vi "提示信息.vi"(0 "LstBox引用句柄":refnum<vi>, 1 "截取数组大小":dbl, 2 "保留行数":dbl, 5 "旧信息":string[](array[string]), 7 "新信息":string, 11 "error in (no error)":errorcluster caption="错误输入（无错误）") -> (4 "引用输出":refnum<vi>, 15 "error out":errorcluster caption="错误输出")   [LabVIEW 2019]
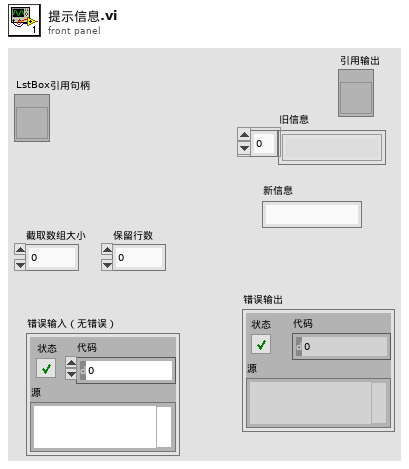
[diagram p1: front panel]
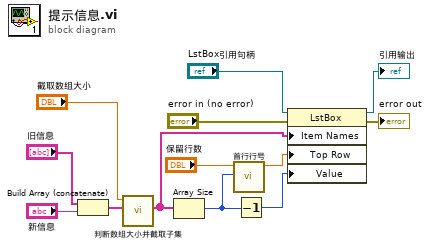
[diagram p0: block diagram]
diagram:
  n1 = Build Array (concatenate)("旧信息", "新信息") -> (w10:string[])
  n2 = call "判断数组大小并截取子集.vi"("数组"=w10, "截取数组大小"="截取数组大小") -> ("输出数组"=w7:string[])  [unwired: 9 in]
  n3 = Array Size(array=w7) -> (size(s)=w6:i32)
  n4 = call "首行行号.vi"("原始行"=w6, "保留行数"="保留行数") -> ("新行"=w4:dbl)  [unwired: 9 in]
  n5 = Decrement(x=w6) -> (x-1=w5:i32)
  n6 = property class="LstBox"(reference="LstBox引用句柄", error in="error in (no error)", "Item Names"=w7, "Top Row"=w4, "Value"=w5) -> (reference out=→"引用输出":refnum<vi>, error out=→"error out":errorcluster)
